vi "Tosca-Test Compound Logic.vi"() -> ()   [LabVIEW 2015]
panel:
  out "ANDs":bool[](array[boolean])
  out "logical OR":bool
  in  "Array":bool[](array[boolean])
  in  "Operator":enum16{"AND", "OR"}[](array[ring])
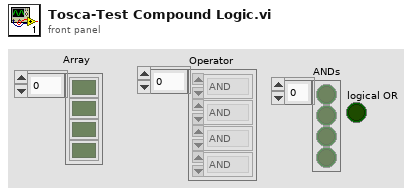
[diagram p1: front panel]
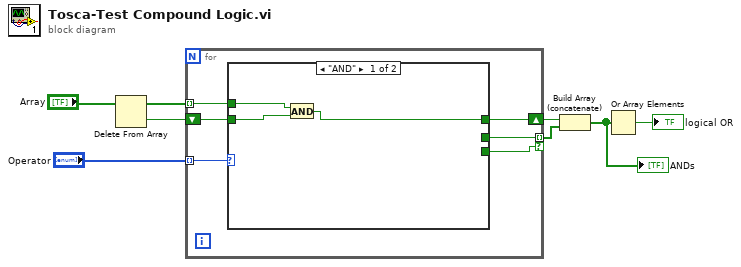
[diagram p0: block diagram]
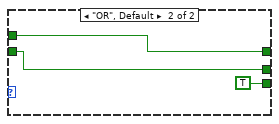
[diagram p2: hidden frame]
diagram:
  n1 = Delete From Array(array="Array") -> (deleted portion=w6:bool, array with subset deleted=w5:bool[])  [unwired: 2 in]
  n2 = for {
    tunnel: "Operator" -> [w14] mode=indexing
    shift-right: [w11] -> w3
    shift-left: w6 -> [w12]
    tunnel: w5 -> [w13] mode=indexing
    tunnel: [w10] -> w2 mode=indexing if=w9
    n3 = case shown="\"AND\"" w14 {
      tunnel: w13 -> [w16 w20]
      tunnel: w12 -> [w17 w19]
      tunnel: [w15 w20] -> w11
      tunnel: [_ w19] -> w10
      tunnel: [_ TRUE] -> w9
      frame "AND" {
        n4 = And(x=w16, y=w17) -> (x .and. y?=w15:bool)
      }
      frame "OR", Default {
      }
    }
  }
  n5 = Build Array (concatenate)(w3, w2) -> (w1:bool[])
  "ANDs" <- w1
  n6 = Or Array Elements(Boolean array=w1) -> (logical OR=→"logical OR":bool)
